vi "Set Icon Text Constant.vi"(8 "error in":errorcluster, 10 "Text":string, 11 "VI in":refnum<vi>) -> (0 "error out":errorcluster, 3 "VI out":refnum<vi>)   [LabVIEW 2020, in "ConstantErrorsMaker.lvlib"]
uses:
  <vilib>/LabVIEW Icon API/API_Text.ctl
  ConstantErrorsMaker.lvlib
  <vilib>/LabVIEW Icon API/LabVIEW Icon API.lvlib
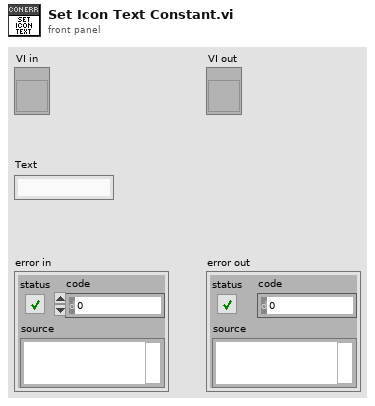
[diagram p1: front panel]
types:
  T1 = typedef "LabVIEW Icon API.lvlib/API_Text.ctl" = cluster{"Line 1 text":string, "Line 2 text":string, "Line 3 text":string, "Line 4 text":string}
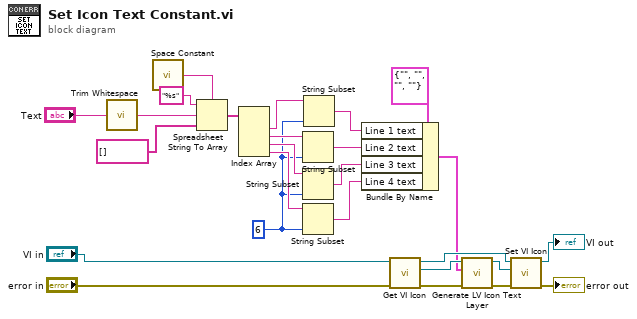
[diagram p0: block diagram]
diagram:
  w2 = 6 ("length (rest)")
  n1 = call <vilib>:"Trim Whitespace.vi"("string"="Text") -> ("trimmed string"=w20:string)  [unwired: 1 in]
  n2 = call <vilib>:"Space Constant.vi"() -> ("String"=w18:string)
  n3 = Spreadsheet String To Array(delimiter (Tab)=w18, format string="%s", spreadsheet string=w20, array type (2D Dbl)=string[] [] ("format string")) -> (array=w16:string[])
  n4 = Index Array(array=w16) -> (element #1=w15:string, element #2=w14:string, element #3=w13:string, element #4=w4:string)  [unwired: 4 in]
  n5 = String Subset(string=w14, length (rest)=w2) -> (substring=w11:string)  [unwired: 1 in]
  n6 = String Subset(string=w13, length (rest)=w2) -> (substring=w3:string)  [unwired: 1 in]
  n7 = String Subset(string=w4, length (rest)=w2) -> (substring=w1:string)  [unwired: 1 in]
  n8 = String Subset(string=w15, length (rest)=w2) -> (substring=w12:string)  [unwired: 1 in]
  n9 = Bundle By Name(cluster=T1 {"Line 1 text"="", "Line 2 text"="", "Line 3 text"="", "Line 4 text"=""} ("Text"), "Line 1 text"=w12, "Line 2 text"=w11, "Line 3 text"=w3, "Line 4 text"=w1) -> (w5:T1)
  n10 = call <vilib>:"Get VI Icon.vi"("error in (no error)"="error in", "VI Refnum in"="VI in") -> ("error out"=w24:errorcluster, "Icon"=w7:refnum<class "Icon.lvclass">, "VI Refnum out"=w9:refnum<vi>)  [unwired: 7 in]
  n11 = call <vilib>:"Generate LV Icon Text Layer.vi"("error in (no error)"=w24, "Text"=w5, "Icon in"=w7) -> ("error out"=w23:errorcluster, "Icon out"=w6:refnum<class "Icon.lvclass">)  [unwired: 7 in]
  n12 = call <vilib>:"Set VI Icon.vi"("error in (no error)"=w23, "Icon"=w6, "VI Refnum in"=w9) -> ("error out"=→"error out":errorcluster, "VI Refnum out"=→"VI out":refnum<vi>)  [unwired: 7 in]
